vi "ExcuteSCPICmd.vi"(7 "VISAOperation":T1=enum."OpenDebugPanel", 8 "error in (no error)":errorcluster, 10 "Run Command":string, 11 "VISA resource name":refnum<visa-resource-name>) -> (0 "error out":errorcluster, 1 "Error Response":string, 2 "Results":string, 3 "reference out":refnum<visa-resource-name>)   [LabVIEW 2015]
uses:
  VISAOperation.ctl
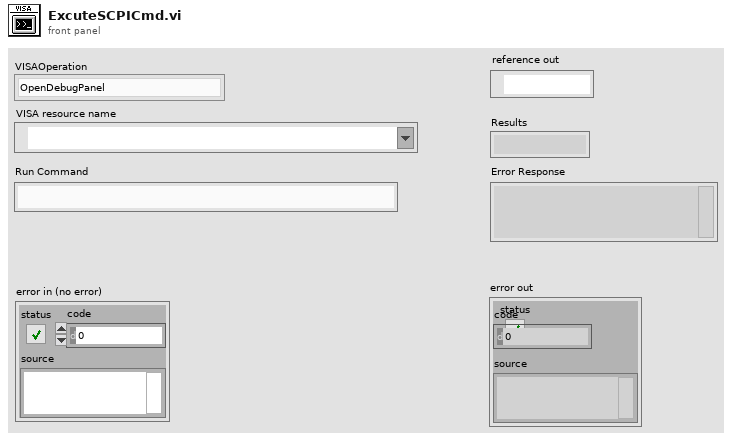
[diagram p1: front panel]
types:
  T1 = typedef "VISAOperation.ctl" = enum16{"RunFile", "OpenDebugPanel", "ReadError", "ReadSTB", "Reset", "Clean", "CloseVISA", "RunCMD", "OpenVISA"}
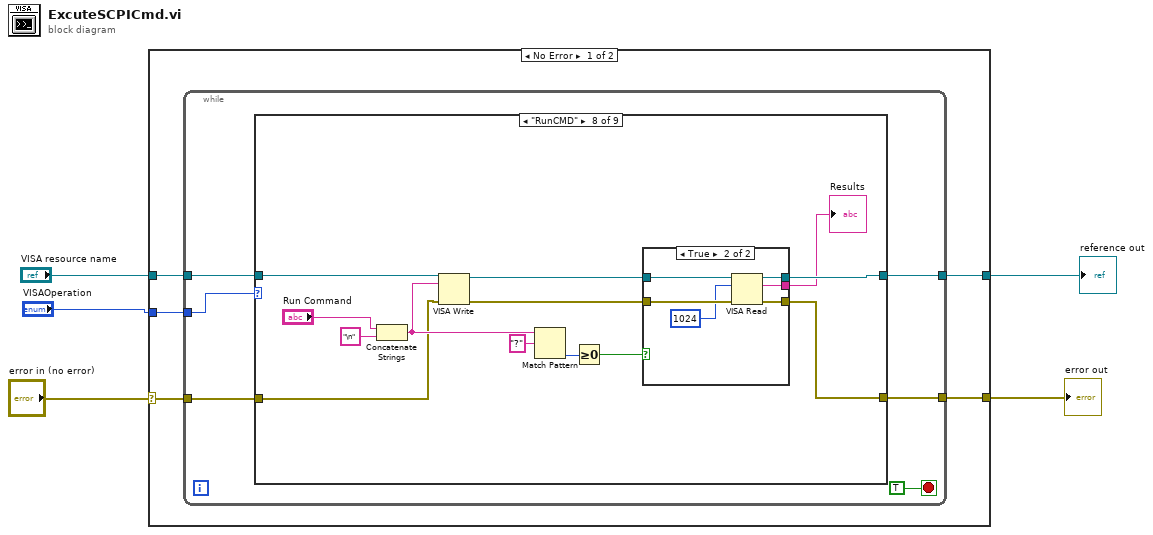
[diagram p0: block diagram]
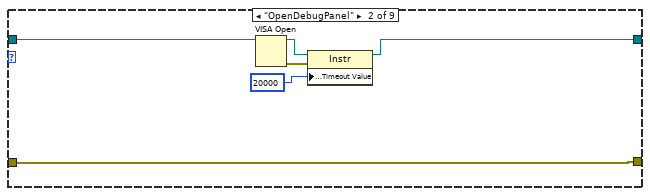
[diagram p3: hidden frame]
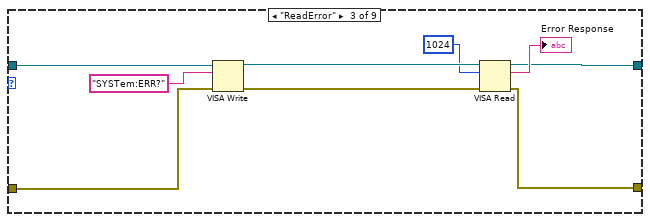
[diagram p4: hidden frame]
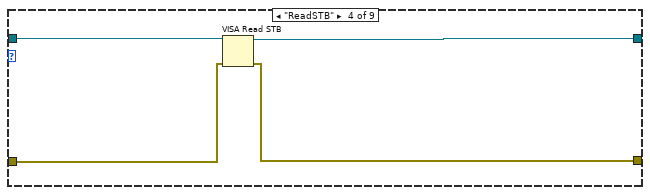
[diagram p5: hidden frame]
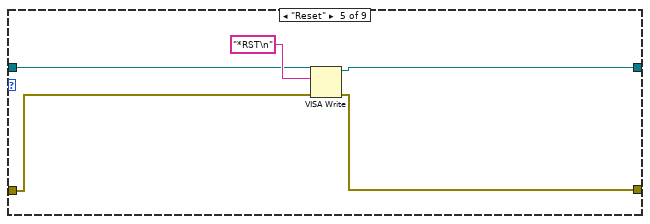
[diagram p6: hidden frame]
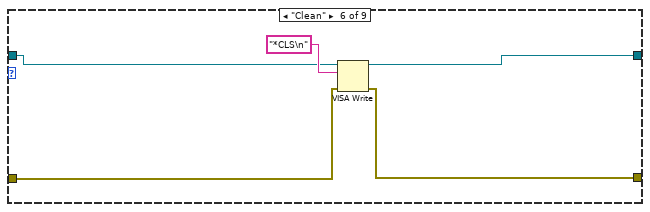
[diagram p7: hidden frame]
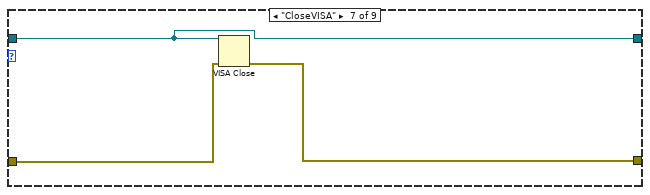
[diagram p8: hidden frame]
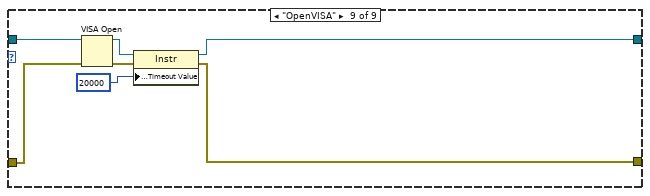
[diagram p10: hidden frame]
diagram:
  n1 = case shown="No Error" "error in (no error)" {
    selector: "error in (no error)" -> [w6 w80]
    tunnel: "VISA resource name" -> [w10 w79]
    tunnel: "VISAOperation" -> [w9 _]
    tunnel: [w8 w79] -> w3
    tunnel: [w7 w80] -> w2
    frame No Error {
      n2 = while {
        tunnel: w10 -> [w15]
        tunnel: w9 -> [w14]
        tunnel: [w13] -> w8
        tunnel: [w12] -> w7
        tunnel: w6 -> [w11]
        stop <- TRUE stop-if-true
        n3 = case shown="\"RunCMD\"" w14 {
          tunnel: w15 -> [w18 w21 w28 w37 w41 w46 w48 w55 w76]
          tunnel: [w18 w20 w27 w36 w40 w45 w48 w54 w75] -> w13
          tunnel: w11 -> [w17 w19 w26 w35 w39 w44 w50 w53 w74]
          tunnel: [w17 w19 w25 w34 w38 w43 w49 w52 w73] -> w12
          frame "RunFile", Default {
          }
          frame "OpenDebugPanel" {
            n4 = VISA Open(VISA resource name=w21) -> (VISA resource name=w22:refnum<visa-resource-name>, error out=w23:errorcluster)  [unwired: 4 in]
            n5 = property class="Instr"(reference=w22, error in=w23, "General Settings:Timeout Value"=u32 20000) -> (reference out=w20:refnum<visa-resource-name>)  [unwired: 1 out]
          }
          frame "ReadError" {
            n6 = VISA Write(VISA resource name=w28, write buffer="SYSTem:ERR?", error in (no error)=w26) -> (VISA resource name out=w32:refnum<visa-resource-name>, error out=w31:errorcluster)  [unwired: 1 out]
            n7 = VISA Read(VISA resource name=w32, byte count=u32 1024, error in (no error)=w31) -> (VISA resource name out=w27:refnum<visa-resource-name>, read buffer=→"Error Response":string, error out=w25:errorcluster)  [unwired: 1 out]
          }
          frame "ReadSTB" {
            n8 = VISA Read STB(8:w35, 11:w37) -> (0:w34:errorcluster, 3:w36:refnum<visa-resource-name>)  [unwired: 1 out]
          }
          frame "Reset" {
            n9 = VISA Write(VISA resource name=w41, write buffer="*RST\n", error in (no error)=w39) -> (VISA resource name out=w40:refnum<visa-resource-name>, error out=w38:errorcluster)  [unwired: 1 out]
          }
          frame "Clean" {
            n10 = VISA Write(VISA resource name=w46, write buffer="*CLS\n", error in (no error)=w44) -> (VISA resource name out=w45:refnum<visa-resource-name>, error out=w43:errorcluster)  [unwired: 1 out]
          }
          frame "CloseVISA" {
            n11 = VISA Close(VISA resource name=w48, error in (no error)=w50) -> (error out=w49:errorcluster)
          }
          frame "RunCMD" {
            n12 = Concatenate Strings("Run Command", "\n" ("write buffer")) -> (w56:string)
            n13 = VISA Write(VISA resource name=w55, write buffer=w56, error in (no error)=w53) -> (VISA resource name out=w58:refnum<visa-resource-name>, error out=w57:errorcluster)  [unwired: 1 out]
            n14 = Match Pattern(string=w56, regular expression="?") -> (offset past match=w60:i32)  [unwired: 1 in, 3 out]
            n15 = Greater Or Equal To 0?(x=w60) -> (x >= 0?=w59:bool)
            n16 = case shown="True" w59 {
              tunnel: w58 -> [w65 w71]
              tunnel: w57 -> [w64 w70]
              tunnel: [w65 w68] -> w54
              tunnel: [w64 w67] -> w52
              tunnel: [_ w66] -> w51
              frame False {
              }
              frame True {
                n17 = VISA Read(VISA resource name=w71, byte count=u32 1024, error in (no error)=w70) -> (VISA resource name out=w68:refnum<visa-resource-name>, read buffer=w66:string, error out=w67:errorcluster)  [unwired: 1 out]
              }
            }
            "Results" <- w51
          }
          frame "OpenVISA" {
            n18 = VISA Open(error in (no error)=w74, VISA resource name=w76) -> (VISA resource name=w72:refnum<visa-resource-name>, error out=w77:errorcluster)  [unwired: 3 in]
            n19 = property class="Instr"(reference=w72, error in=w77, "General Settings:Timeout Value"=u32 20000) -> (reference out=w75:refnum<visa-resource-name>, error out=w73:errorcluster)
          }
        }
      }
    }
    frame Error {
    }
  }
  "reference out" <- w3
  "error out" <- w2
